vi "String To Variant.vi"(4 "Type Enum [auto]":T1, 5 "Strip Whitespace? [T]":bool=TRUE, 6 "Variant Type\\default":variant, 7 "Name (error)":string, 8 "error in (no error)":errorcluster, 9 "Use LV Default? [F]":bool, 10 "String":string, 11 "Registry Object":refnum<class "Carya Config.lvclass">) -> (0 "error out":errorcluster, 2 "Variant":variant, 3 "Registry Object":refnum<class "Carya Config.lvclass">)   [LabVIEW 2013, in "Carya Config.lvclass"]
doc: "Copyright 2018, Carya Automatisering, Wiebe Walstra."
uses:
  Carya Config.lvclass
  <vilib>/Utility/VariantDataType/Type.ctl
  <vilib>/Utility/error.llb/Error Cluster From Error Code.vi
  <vilib>/ErrorRing/Error Ring.xnode
  <vilib>/Utility/VariantDataType/VariantType.lvlib
  CConfig Variant Accessor/CConfig Variant Accessor.lvclass
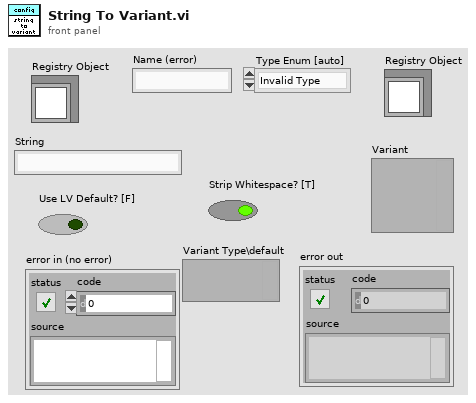
[diagram p1: front panel]
types:
  T1 = typedef "VariantType.lvlib/Type.ctl" = enum8{"Invalid Type", "Void", "I8", "I16", "I32", "I64", "U8", "U16", "U32", "U64", "Single Float", "Double Float", "Extended Float", "Single Complex", "Double Complex", "Extended Complex", "Enum U8", "Enum U16", "Enum U32", "Enum U64", "Single Float With Unit", "Double Float With Unit", "Extended Float With Unit", "Single Complex with Unit", "Double Complex with Unit", "Extended Complex with Unit", "Boolean", "String", "Path", "Picture", "Tag", "Array", "Cluster", "Variant", "LV Variant", "Waveform", "Timestamp", "Digital Waveform", "Digital Data", "ExpressData", "Refnum", "External Data", "VI", "Poly VI", "LabVIEW Class Instance", "Fixed Point"}
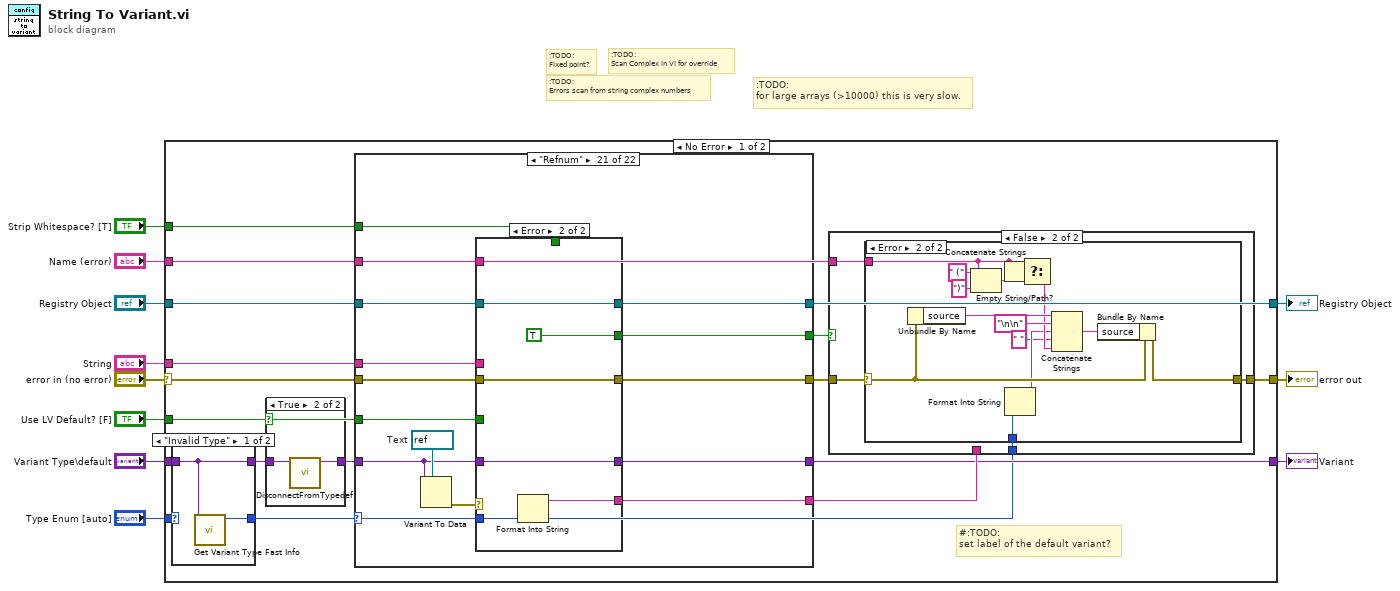
[diagram p0: block diagram]
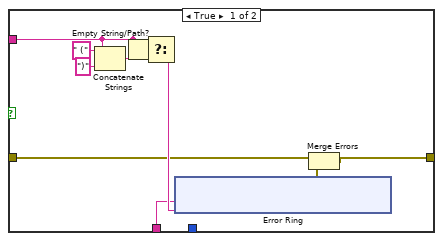
[diagram p2: hidden frame]
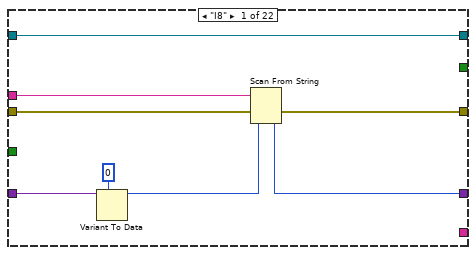
[diagram p6: hidden frame]
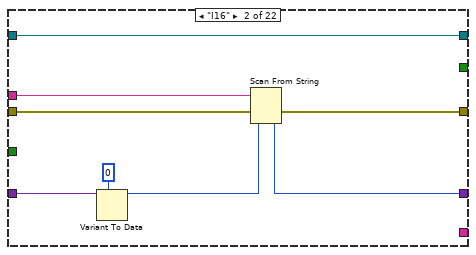
[diagram p7: hidden frame]
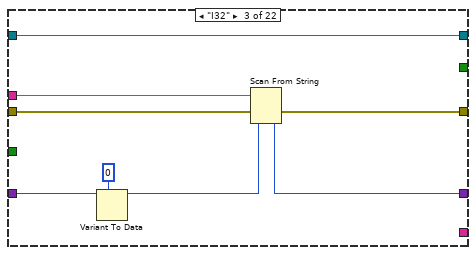
[diagram p8: hidden frame]
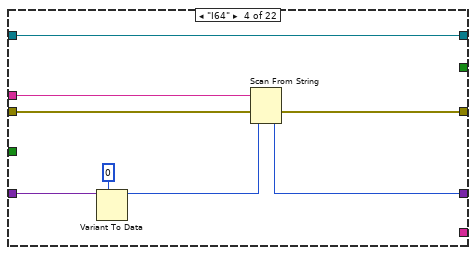
[diagram p9: hidden frame]
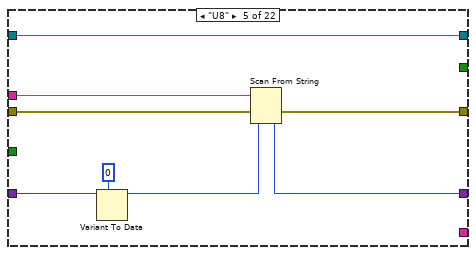
[diagram p10: hidden frame]
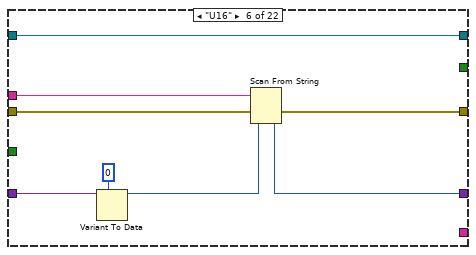
[diagram p11: hidden frame]
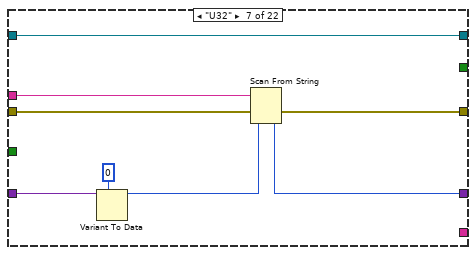
[diagram p12: hidden frame]
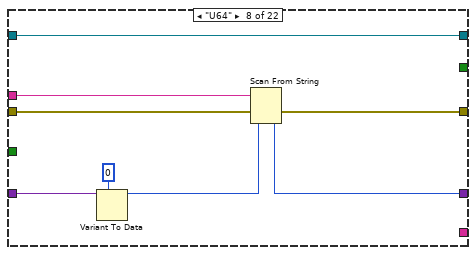
[diagram p13: hidden frame]
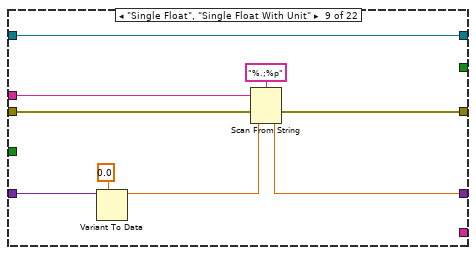
[diagram p14: hidden frame]
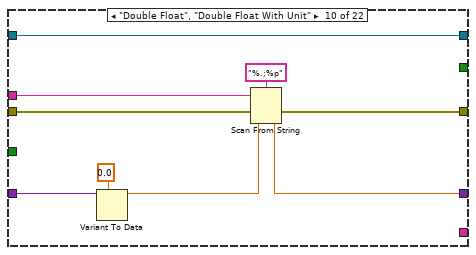
[diagram p15: hidden frame]
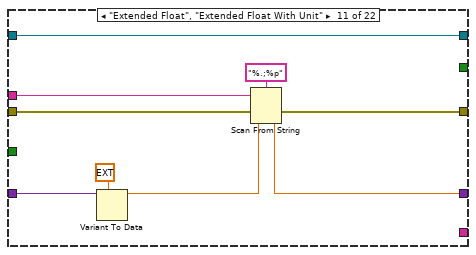
[diagram p16: hidden frame]
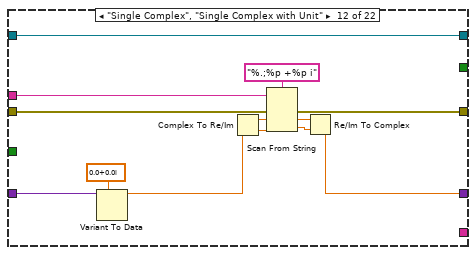
[diagram p17: hidden frame]
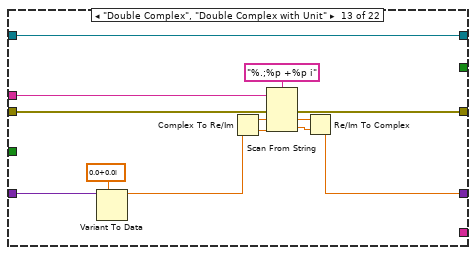
[diagram p18: hidden frame]
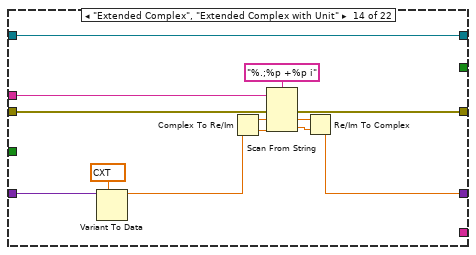
[diagram p19: hidden frame]
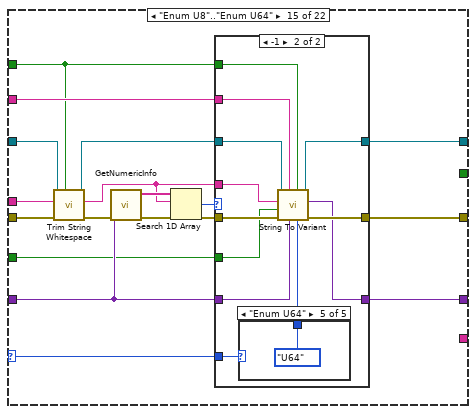
[diagram p20: hidden frame]
diagram:
  # ":TODO:\nfor large arrays (>10000) this is very slow."
  # ":TODO:\nScan Complex in VI for override"
  # ":TODO:\nErrors scan from string complex numbers"
  # ":TODO:\nFixed point?"
  n1 = case shown="No Error" "error in (no error)" {
    selector: "error in (no error)" -> [w15 w648]
    tunnel: "String" -> [w12 _]
    tunnel: "Registry Object" -> [w28 w649]
    tunnel: [w27 w649] -> w9
    tunnel: "Type Enum [auto]" -> [w26 _]
    tunnel: "Strip Whitespace? [T]" -> [w23 _]
    tunnel: "Name (error)" -> [w21 _]
    tunnel: "Use LV Default? [F]" -> [w18 _]
    tunnel: "Variant Type\\default" -> [w17 w647]
    tunnel: [w16 w647] -> w3
    tunnel: [w14 w648] -> w1
    frame No Error {
      # "#:TODO:\nset label of the default variant?"
      n2 = case shown="\"Invalid Type\"" w26 {
        selector: w26 -> [_ w72]
        tunnel: w17 -> [w69 w71]
        tunnel: [w70 w72] -> w13
        tunnel: [w69 w71] -> w24
        frame "Invalid Type" {
          n3 = call "Get Variant Type Fast Info.vi"("Variant"=w69) -> ("Type Enum"=w70:T1)  [unwired: 6 in, 4 out]
        }
        frame Default {
        }
      }
      n4 = case shown="True" w18 {
        tunnel: [w66 w68] -> w25
        tunnel: w24 -> [w66 w67]
        frame False {
        }
        frame True {
          n5 = call <vilib>:"DisconnectFromTypedef.vi"("lvvar in"=w67) -> ("lvvar out"=w68:variant)  [unwired: 4 in, 1 out]
        }
      }
      n6 = case shown="\"Refnum\"" w13 {
        selector: w13 -> [_ _ _ _ _ _ _ _ _ _ _ _ _ _ w210 _ _ _ _ _ w622 w642]
        tunnel: [w78 w86 w94 w102 w109 w117 w125 w133 w143 w151 w160 w173 w186 w199 w216 w257 w285 w293 w307 w605 w617 w645] -> w22
        tunnel: w15 -> [w74 w82 w90 w98 w110 w118 w126 w134 w140 w152 w161 w174 w187 w200 w218 w260 w287 w294 w308 w608 w618 w645]
        tunnel: w25 -> [w80 w88 w96 w104 w112 w120 w128 w136 w145 w154 w163 w176 w189 w202 w213 w263 _ w296 w305 _ w616 w646]
        tunnel: w21 -> [_ _ _ _ _ _ _ _ _ _ _ _ _ _ w215 _ _ _ w306 _ w610 _]
        tunnel: [w76 w84 w92 w100 w107 w115 w123 w131 w141 w149 w158 w172 w177 w190 w212 w259 w275 w288 w303 w607 w615 w646] -> w16
        tunnel: w12 -> [w75 w83 w91 w99 w106 w114 w122 w130 w139 w148 w157 w170 w184 w197 w206 w256 w283 w292 w302 w604 w612 _]
        tunnel: w28 -> [w73 w81 w89 w97 w105 w113 w121 w129 w138 w147 w156 w169 w183 w196 w208 w261 w282 w291 w301 w603 w614 w644]
        tunnel: [w73 w81 w89 w97 w105 w113 w121 w129 w138 w147 w156 w169 w183 w196 w214 w261 w286 w290 w300 w606 w613 w644] -> w27
        tunnel: w23 -> [_ _ _ _ _ _ _ _ _ _ _ _ _ _ w204 _ w276 _ w298 _ w609 _]
        tunnel: [_ _ _ _ _ _ _ _ _ _ _ _ _ _ _ _ _ _ _ _ w623 TRUE] -> w20
        tunnel: [_ _ _ _ _ _ _ _ _ _ _ _ _ _ _ _ _ _ _ _ w621 w641] -> w19
        tunnel: w18 -> [_ _ _ _ _ _ _ _ _ _ _ _ _ _ w203 _ _ _ w297 _ w611 _]
        frame "I8" {
          n7 = Variant To Data(type=i8 0, Variant=w80) -> (data=w77:i8)  [unwired: 1 in, 1 out]
          n8 = Scan From String(input string=w75, error in=w74, default 1=w77) -> (error out=w78:errorcluster, output 1=w76:i8)  [unwired: 2 in, 2 out]
        }
        frame "I16" {
          n9 = Variant To Data(type=i16 0, Variant=w88) -> (data=w85:i16)  [unwired: 1 in, 1 out]
          n10 = Scan From String(input string=w83, error in=w82, default 1=w85) -> (error out=w86:errorcluster, output 1=w84:i16)  [unwired: 2 in, 2 out]
        }
        frame "I32" {
          n11 = Variant To Data(type=0, Variant=w96) -> (data=w93:i32)  [unwired: 1 in, 1 out]
          n12 = Scan From String(input string=w91, error in=w90, default 1=w93) -> (error out=w94:errorcluster, output 1=w92:i32)  [unwired: 2 in, 2 out]
        }
        frame "I64" {
          n13 = Variant To Data(type=i64 0, Variant=w104) -> (data=w101:i64)  [unwired: 1 in, 1 out]
          n14 = Scan From String(input string=w99, error in=w98, default 1=w101) -> (error out=w102:errorcluster, output 1=w100:i64)  [unwired: 2 in, 2 out]
        }
        frame "U8" {
          n15 = Variant To Data(type=u8 0, Variant=w112) -> (data=w108:u8)  [unwired: 1 in, 1 out]
          n16 = Scan From String(input string=w106, error in=w110, default 1=w108) -> (error out=w109:errorcluster, output 1=w107:u8)  [unwired: 2 in, 2 out]
        }
        frame "U16" {
          n17 = Variant To Data(type=u16 0, Variant=w120) -> (data=w116:u16)  [unwired: 1 in, 1 out]
          n18 = Scan From String(input string=w114, error in=w118, default 1=w116) -> (error out=w117:errorcluster, output 1=w115:u16)  [unwired: 2 in, 2 out]
        }
        frame "U32" {
          n19 = Variant To Data(type=u32 0, Variant=w128) -> (data=w124:u32)  [unwired: 1 in, 1 out]
          n20 = Scan From String(input string=w122, error in=w126, default 1=w124) -> (error out=w125:errorcluster, output 1=w123:u32)  [unwired: 2 in, 2 out]
        }
        frame "U64" {
          n21 = Variant To Data(type=u64 0, Variant=w136) -> (data=w132:u64)  [unwired: 1 in, 1 out]
          n22 = Scan From String(input string=w130, error in=w134, default 1=w132) -> (error out=w133:errorcluster, output 1=w131:u64)  [unwired: 2 in, 2 out]
        }
        frame "Single Float", "Single Float With Unit" {
          n23 = Variant To Data(type=sgl 0.0, Variant=w145) -> (data=w142:sgl)  [unwired: 1 in, 1 out]
          n24 = Scan From String(format string="%.;%p", input string=w139, error in=w140, default 1=w142) -> (error out=w143:errorcluster, output 1=w141:sgl)  [unwired: 1 in, 2 out]
        }
        frame "Double Float", "Double Float With Unit" {
          n25 = Variant To Data(type=0.0, Variant=w154) -> (data=w150:dbl)  [unwired: 1 in, 1 out]
          n26 = Scan From String(format string="%.;%p", input string=w148, error in=w152, default 1=w150) -> (error out=w151:errorcluster, output 1=w149:dbl)  [unwired: 1 in, 2 out]
        }
        frame "Extended Float", "Extended Float With Unit" {
          n27 = Variant To Data(type=ext 0.0, Variant=w163) -> (data=w159:ext)  [unwired: 1 in, 1 out]
          n28 = Scan From String(format string="%.;%p", input string=w157, error in=w161, default 1=w159) -> (error out=w160:errorcluster, output 1=w158:ext)  [unwired: 1 in, 2 out]
        }
        frame "Single Complex", "Single Complex with Unit" {
          n29 = Variant To Data(type=csg 0.0+0.0i, Variant=w176) -> (data=w171:csg)  [unwired: 1 in, 1 out]
          n30 = Complex To Re/Im(x + iy=w171) -> (x=w167:sgl, y=w166:sgl)
          n31 = Scan From String(format string="%.;%p +%p i", input string=w170, error in=w174, default 1=w167, default 2=w166) -> (error out=w173:errorcluster, output 1=w165:sgl, output 2=w164:sgl)  [unwired: 1 in, 2 out]
          n32 = Re/Im To Complex(1:w164, 2:w165) -> (0:w172:csg)
        }
        frame "Double Complex", "Double Complex with Unit" {
          n33 = Variant To Data(type=cdb 0.0+0.0i, Variant=w189) -> (data=w185:cdb)  [unwired: 1 in, 1 out]
          n34 = Complex To Re/Im(x + iy=w185) -> (x=w181:dbl, y=w180:dbl)
          n35 = Scan From String(format string="%.;%p +%p i", input string=w184, error in=w187, default 1=w181, default 2=w180) -> (error out=w186:errorcluster, output 1=w179:dbl, output 2=w178:dbl)  [unwired: 1 in, 2 out]
          n36 = Re/Im To Complex(1:w178, 2:w179) -> (0:w177:cdb)
        }
        frame "Extended Complex", "Extended Complex with Unit" {
          n37 = Variant To Data(type=cxt 0.0+0.0i, Variant=w202) -> (data=w198:cxt)  [unwired: 1 in, 1 out]
          n38 = Complex To Re/Im(x + iy=w198) -> (x=w194:ext, y=w193:ext)
          n39 = Scan From String(format string="%.;%p +%p i", input string=w197, error in=w200, default 1=w194, default 2=w193) -> (error out=w199:errorcluster, output 1=w192:ext, output 2=w191:ext)  [unwired: 1 in, 2 out]
          n40 = Re/Im To Complex(1:w191, 2:w192) -> (0:w190:cxt)
        }
        frame "Enum U8".."Enum U64" {
          n41 = call-dynamic "Trim String Whitespace.vi"("Strip Whitespace? [T]"=w204, "error in (no error)"=w218, "String"=w206, "Registry Object"=w208) -> ("error out"=w209:errorcluster, "Trimmed string"=w205:string, "Registry Object"=w207:refnum<class "Carya Config.lvclass">)  [unwired: 5 in]
          n42 = call <vilib>:"GetNumericInfo.vi"("error in (no error)"=w209, "Variant"=w213) -> ("error out"=w217:errorcluster, "EnumNames"=w219:string[])  [unwired: 6 in, 2 out]
          n43 = Search 1D Array(1D array=w219, element=w205) -> (index of element=w211:i32)  [unwired: 1 in]
          n44 = case shown="-1" w211 {
            selector: w211 -> [w222 _]
            tunnel: w217 -> [w223 w249]
            tunnel: [w223 w248] -> w216
            tunnel: w215 -> [_ w247]
            tunnel: w207 -> [w224 w246]
            tunnel: [w224 w245] -> w214
            tunnel: w213 -> [_ w244]
            tunnel: [w221 w243] -> w212
            tunnel: w205 -> [_ w242]
            tunnel: w210 -> [w220 w241]
            tunnel: w204 -> [_ w239]
            tunnel: w203 -> [_ w238]
            frame Default {
              n45 = case shown="\"Enum U8\"" w220 {
                tunnel: w222 -> [_ w228 w231 w234 w237]
                tunnel: [variant ("lvvar out") w227 w230 w233 w236] -> w221
                frame Default {
                }
                frame "Enum U8" {
                  n46 = Variant To Data(type=u8 0, Variant=w228) -> (data=w227:u8)  [unwired: 1 in, 1 out]
                }
                frame "Enum U16" {
                  n47 = Variant To Data(type=u16 0, Variant=w231) -> (data=w230:u16)  [unwired: 1 in, 1 out]
                }
                frame "Enum U32" {
                  n48 = Variant To Data(type=u32 0, Variant=w234) -> (data=w233:u32)  [unwired: 1 in, 1 out]
                }
                frame "Enum U64" {
                  n49 = Variant To Data(type=u64 0, Variant=w237) -> (data=w236:u64)  [unwired: 1 in, 1 out]
                }
              }
            }
            frame -1 {
              n50 = case shown="\"Enum U64\"" w241 {
                tunnel: [_ Type."U8" ("Type Enum [auto]") Type."U16" ("Type Enum [auto]") Type."U32" ("Type Enum [auto]") Type."U64" ("Type Enum [auto]")] -> w240
                frame Default {
                }
                frame "Enum U8" {
                }
                frame "Enum U16" {
                }
                frame "Enum U32" {
                }
                frame "Enum U64" {
                }
              }
              n51 = call-dynamic "String To Variant.vi"("Type Enum [auto]"=w240, "Strip Whitespace? [T]"=w239, "Variant Type\\default"=w244, "Name (error)"=w247, "error in (no error)"=w249, "Use LV Default? [F]"=w238, "String"=w242, "Registry Object"=w246) -> ("error out"=w248:errorcluster, "Variant"=w243:variant, "Registry Object"=w245:refnum<class "Carya Config.lvclass">)  [unwired: 1 in]
            }
          }
        }
        frame "Boolean" {
          # "false, true\nF, T\nFALSE, TRUE\n0, 1\nY, N\nYes, No\nYES, NO"
          n52 = Variant To Data(type=TRUE, Variant=w263) -> (data=w258:bool)  [unwired: 1 in, 1 out]
          n53 = Decimal String To Number(string=w256, default (0L)=0 ("default (0 I32)")) -> (offset past number=w254:i32)  [unwired: 1 in, 1 out]
          n54 = case shown="1.." w254 {
            tunnel: w260 -> [w269 w274]
            tunnel: [w268 w273] -> w259
            tunnel: w258 -> [w267 w272]
            tunnel: [w266 w271] -> w257
            tunnel: w256 -> [w265 w270]
            frame 1.. {
              n55 = Scan From String(format string="%d", input string=w265, error in=w269, default 1=w267) -> (error out=w266:errorcluster, output 1=w268:bool)  [unwired: 1 in, 2 out]
            }
            frame Default {
              n56 = Scan From String(input string=w270, error in=w274, default 1=w272) -> (error out=w271:errorcluster, output 1=w273:bool)  [unwired: 2 in, 2 out]
            }
          }
        }
        frame "String" {
          n57 = call-dynamic "String (RAW) To String.vi"("error in (no error)"=w287, "String (RAW)"=w283, "Registry Object"=w282) -> ("error out"=w284:errorcluster, "String"=w278:string, "Registry Object"=w280:refnum<class "Carya Config.lvclass">)  [unwired: 6 in]
          n58 = call-dynamic "Trim String Whitespace.vi"("Strip Whitespace? [T]"=w276, "error in (no error)"=w284, "String"=w278, "Registry Object"=w280) -> ("error out"=w281:errorcluster, "Trimmed string"=w277:string, "Registry Object"=w279:refnum<class "Carya Config.lvclass">)  [unwired: 5 in]
          n59 = call-dynamic "Unescape String.vi"("error in (no error)"=w281, "String"=w277, "Registry Object"=w279) -> ("error out"=w285:errorcluster, "Unescaped string"=w275:string, "Registry Object"=w286:refnum<class "Carya Config.lvclass">)  [unwired: 6 in]
        }
        frame "Path" {
          n60 = Variant To Data(type=path "", Variant=w296) -> (data=w289:path)  [unwired: 1 in, 1 out]
          n61 = call-dynamic "String To Path.vi"("Default"=w289, "error in (no error)"=w294, "String"=w292, "Registry Object"=w291) -> ("error out"=w293:errorcluster, "Path"=w288:path, "Registry Object"=w290:refnum<class "Carya Config.lvclass">)  [unwired: 5 in]
        }
        frame "Array" {
          n62 = call <vilib>:"GetArrayInfo.vi"("Variant"=w305) -> ("ArrayElement"=w299:variant, "NDims"=w304:i32)  [unwired: 7 in, 2 out]
          n63 = case shown="1" w304 {
            selector: w304 -> [w314 _]
            tunnel: w308 -> [w315 w332]
            tunnel: [w312 w335] -> w307
            tunnel: w306 -> [w313 w329]
            tunnel: w305 -> [w309 w327]
            tunnel: [w309 w334] -> w303
            tunnel: w302 -> [_ w333]
            tunnel: w301 -> [w310 w331]
            tunnel: [w310 w330] -> w300
            tunnel: w299 -> [_ w326]
            tunnel: w298 -> [_ w325]
            tunnel: w297 -> [_ w324]
            frame Default {
              n64 = xnode "Error Ring"("parameter 0"=w314, "parameter 1"=w313) -> ("error out"=w311:errorcluster)
              n65 = Merge Errors(w315, w311) -> (w312:errorcluster)
            }
            frame 1 {
              n66 = call "Get Variant Type Fast Info.vi"("Variant"=w326) -> ("Type Enum"=w328:T1)  [unwired: 6 in, 4 out]
              n67 = case shown="Default" w328 {
                selector: w328 -> [_ _ _ _ _ _ _ _ _ _ _ _ _ w586]
                tunnel: [w336 w355 w374 w393 w412 w431 w450 w469 w494 w500 w519 w538 w558 w583] -> w335
                tunnel: [w346 w365 w384 w403 w422 w441 w460 w479 w497 w510 w529 w548 w557 w581] -> w334
                tunnel: w333 -> [w344 w363 w382 w401 w420 w439 w458 w477 w488 w508 w527 w546 w561 w576]
                tunnel: w332 -> [w337 w356 w375 w394 w413 w432 w451 w470 w495 w501 w520 w539 w560 w589]
                tunnel: w331 -> [w345 w364 w383 w402 w421 w440 w459 w478 w493 w509 w528 w547 w562 w574]
                tunnel: [w345 w364 w383 w402 w421 w440 w459 w478 w492 w509 w528 w547 w562 w570] -> w330
                tunnel: w329 -> [_ _ _ _ _ _ _ _ _ _ _ _ _ w588]
                tunnel: w326 -> [_ _ _ _ _ _ _ _ _ _ _ _ _ w587]
                tunnel: w327 -> [w347 w366 w385 w404 w423 w442 w461 w480 w498 w511 w530 w549 w557 w584]
                tunnel: w325 -> [_ _ _ _ _ _ _ _ w491 _ _ _ _ w573]
                tunnel: w324 -> [_ _ _ _ _ _ _ _ _ _ _ _ _ w572]
                frame "I8" {
                  # "we can't use spr. str to array directly to get the type...\nwe'll not notice any errors..."
                  n68 = Spreadsheet String To Array(delimiter (Tab)=",", format string="", spreadsheet string=w344, array type (2D Dbl)=string[] []) -> (array=w340:string[])
                  n69 = for {
                    tunnel: w340 -> [w354] mode=indexing
                    tunnel: [w351] -> w339 mode=indexing
                    shift-right: [w349] -> w336
                    shift-left: w337 -> [w350]
                    n70 = Scan From String(format string="%d", input string=w354, error in=w350, default 1=i8 0 ("default value 1")) -> (error out=w349:errorcluster, output 1=w351:i8)  [unwired: 1 in, 2 out]
                  }
                  n71 = Variant To Flattened String(Variant=w347) -> (1:w348:i16[])  [unwired: 1 out]
                  n72 = Flatten To String(anything=w339) -> (data string=w338:string)  [unwired: 3 in, 2 out]
                  n73 = Flattened String To Variant(6:w338, 7:w348) -> (3:w346:variant)  [unwired: 1 in, 1 out]
                }
                frame "I16" {
                  # "we can't use spr. str to array directly to get the type...\nwe'll not notice any errors..."
                  n74 = Spreadsheet String To Array(delimiter (Tab)=",", format string="", spreadsheet string=w363, array type (2D Dbl)=string[] []) -> (array=w359:string[])
                  n75 = for {
                    tunnel: w359 -> [w373] mode=indexing
                    tunnel: [w370] -> w358 mode=indexing
                    shift-right: [w368] -> w355
                    shift-left: w356 -> [w369]
                    n76 = Scan From String(format string="%d", input string=w373, error in=w369, default 1=i16 0 ("default value 1")) -> (error out=w368:errorcluster, output 1=w370:i16)  [unwired: 1 in, 2 out]
                  }
                  n77 = Variant To Flattened String(Variant=w366) -> (1:w367:i16[])  [unwired: 1 out]
                  n78 = Flatten To String(anything=w358) -> (data string=w357:string)  [unwired: 3 in, 2 out]
                  n79 = Flattened String To Variant(6:w357, 7:w367) -> (3:w365:variant)  [unwired: 1 in, 1 out]
                }
                frame "I32" {
                  # "we can't use spr. str to array directly to get the type...\nwe'll not notice any errors..."
                  n80 = Spreadsheet String To Array(delimiter (Tab)=",", format string="", spreadsheet string=w382, array type (2D Dbl)=string[] []) -> (array=w378:string[])
                  n81 = for {
                    tunnel: w378 -> [w392] mode=indexing
                    tunnel: [w389] -> w377 mode=indexing
                    shift-right: [w387] -> w374
                    shift-left: w375 -> [w388]
                    n82 = Scan From String(format string="%d", input string=w392, error in=w388, default 1=0 ("default value 1")) -> (error out=w387:errorcluster, output 1=w389:i32)  [unwired: 1 in, 2 out]
                  }
                  n83 = Variant To Flattened String(Variant=w385) -> (1:w386:i16[])  [unwired: 1 out]
                  n84 = Flatten To String(anything=w377) -> (data string=w376:string)  [unwired: 3 in, 2 out]
                  n85 = Flattened String To Variant(6:w376, 7:w386) -> (3:w384:variant)  [unwired: 1 in, 1 out]
                }
                frame "I64" {
                  # "we can't use spr. str to array directly to get the type...\nwe'll not notice any errors..."
                  n86 = Spreadsheet String To Array(delimiter (Tab)=",", format string="", spreadsheet string=w401, array type (2D Dbl)=string[] []) -> (array=w397:string[])
                  n87 = for {
                    tunnel: w397 -> [w411] mode=indexing
                    tunnel: [w408] -> w396 mode=indexing
                    shift-right: [w406] -> w393
                    shift-left: w394 -> [w407]
                    n88 = Scan From String(format string="%d", input string=w411, error in=w407, default 1=i64 0 ("default value 1")) -> (error out=w406:errorcluster, output 1=w408:i64)  [unwired: 1 in, 2 out]
                  }
                  n89 = Variant To Flattened String(Variant=w404) -> (1:w405:i16[])  [unwired: 1 out]
                  n90 = Flatten To String(anything=w396) -> (data string=w395:string)  [unwired: 3 in, 2 out]
                  n91 = Flattened String To Variant(6:w395, 7:w405) -> (3:w403:variant)  [unwired: 1 in, 1 out]
                }
                frame "U8" {
                  # "we can't use spr. str to array directly to get the type...\nwe'll not notice any errors..."
                  n92 = Spreadsheet String To Array(delimiter (Tab)=",", format string="", spreadsheet string=w420, array type (2D Dbl)=string[] []) -> (array=w416:string[])
                  n93 = for {
                    tunnel: w416 -> [w430] mode=indexing
                    tunnel: [w427] -> w415 mode=indexing
                    shift-right: [w425] -> w412
                    shift-left: w413 -> [w426]
                    n94 = Scan From String(format string="%d", input string=w430, error in=w426, default 1=u8 0 ("default value 1")) -> (error out=w425:errorcluster, output 1=w427:u8)  [unwired: 1 in, 2 out]
                  }
                  n95 = Variant To Flattened String(Variant=w423) -> (1:w424:i16[])  [unwired: 1 out]
                  n96 = Flatten To String(anything=w415) -> (data string=w414:string)  [unwired: 3 in, 2 out]
                  n97 = Flattened String To Variant(6:w414, 7:w424) -> (3:w422:variant)  [unwired: 1 in, 1 out]
                }
                frame "U16" {
                  # "we can't use spr. str to array directly to get the type...\nwe'll not notice any errors..."
                  n98 = Spreadsheet String To Array(delimiter (Tab)=",", format string="", spreadsheet string=w439, array type (2D Dbl)=string[] []) -> (array=w435:string[])
                  n99 = for {
                    tunnel: w435 -> [w449] mode=indexing
                    tunnel: [w446] -> w434 mode=indexing
                    shift-right: [w444] -> w431
                    shift-left: w432 -> [w445]
                    n100 = Scan From String(format string="%d", input string=w449, error in=w445, default 1=u16 0 ("default value 1")) -> (error out=w444:errorcluster, output 1=w446:u16)  [unwired: 1 in, 2 out]
                  }
                  n101 = Variant To Flattened String(Variant=w442) -> (1:w443:i16[])  [unwired: 1 out]
                  n102 = Flatten To String(anything=w434) -> (data string=w433:string)  [unwired: 3 in, 2 out]
                  n103 = Flattened String To Variant(6:w433, 7:w443) -> (3:w441:variant)  [unwired: 1 in, 1 out]
                }
                frame "U32" {
                  # "we can't use spr. str to array directly to get the type...\nwe'll not notice any errors..."
                  n104 = Spreadsheet String To Array(delimiter (Tab)=",", format string="", spreadsheet string=w458, array type (2D Dbl)=string[] []) -> (array=w454:string[])
                  n105 = for {
                    tunnel: w454 -> [w468] mode=indexing
                    tunnel: [w465] -> w453 mode=indexing
                    shift-right: [w463] -> w450
                    shift-left: w451 -> [w464]
                    n106 = Scan From String(format string="%d", input string=w468, error in=w464, default 1=u32 0 ("default value 1")) -> (error out=w463:errorcluster, output 1=w465:u32)  [unwired: 1 in, 2 out]
                  }
                  n107 = Variant To Flattened String(Variant=w461) -> (1:w462:i16[])  [unwired: 1 out]
                  n108 = Flatten To String(anything=w453) -> (data string=w452:string)  [unwired: 3 in, 2 out]
                  n109 = Flattened String To Variant(6:w452, 7:w462) -> (3:w460:variant)  [unwired: 1 in, 1 out]
                }
                frame "U64" {
                  # "we can't use spr. str to array directly to get the type...\nwe'll not notice any errors..."
                  n110 = Spreadsheet String To Array(delimiter (Tab)=",", format string="", spreadsheet string=w477, array type (2D Dbl)=string[] []) -> (array=w473:string[])
                  n111 = for {
                    tunnel: w473 -> [w487] mode=indexing
                    tunnel: [w484] -> w472 mode=indexing
                    shift-right: [w482] -> w469
                    shift-left: w470 -> [w483]
                    n112 = Scan From String(format string="%d", input string=w487, error in=w483, default 1=u64 0 ("default value 1")) -> (error out=w482:errorcluster, output 1=w484:u64)  [unwired: 1 in, 2 out]
                  }
                  n113 = Variant To Flattened String(Variant=w480) -> (1:w481:i16[])  [unwired: 1 out]
                  n114 = Flatten To String(anything=w472) -> (data string=w471:string)  [unwired: 3 in, 2 out]
                  n115 = Flattened String To Variant(6:w471, 7:w481) -> (3:w479:variant)  [unwired: 1 in, 1 out]
                }
                frame "String" {
                  # "we can't use spr. str to array directly to get the type...\nwe'll not notice any errors..."
                  n116 = call-dynamic "String To Array.vi"("Unescape? [F]"=TRUE, "Strip Whitespace? [T]"=w491, "error in (no error)"=w495, "resulting string"=w488, "Registry Object"=w493) -> ("error out"=w494:errorcluster, "Array"=w489:string[], "Registry Object"=w492:refnum<class "Carya Config.lvclass">)  [unwired: 4 in]
                  n117 = Variant To Flattened String(Variant=w498) -> (1:w499:i16[])  [unwired: 1 out]
                  n118 = Flatten To String(anything=w489) -> (data string=w496:string)  [unwired: 3 in, 2 out]
                  n119 = Flattened String To Variant(6:w496, 7:w499) -> (3:w497:variant)  [unwired: 1 in, 1 out]
                }
                frame "Single Float", "Single Float With Unit" {
                  # "we can't use spr. str to array directly to get the type...\nwe'll not notice any errors..."
                  n120 = Spreadsheet String To Array(delimiter (Tab)=",", format string="", spreadsheet string=w508, array type (2D Dbl)=string[] []) -> (array=w504:string[])
                  n121 = for {
                    tunnel: w504 -> [w518] mode=indexing
                    tunnel: [w515] -> w503 mode=indexing
                    shift-right: [w513] -> w500
                    shift-left: w501 -> [w514]
                    n122 = Scan From String(format string="%.;%p", input string=w518, error in=w514, default 1=sgl 0.0 ("default value 1")) -> (error out=w513:errorcluster, output 1=w515:sgl)  [unwired: 1 in, 2 out]
                  }
                  n123 = Variant To Flattened String(Variant=w511) -> (1:w512:i16[])  [unwired: 1 out]
                  n124 = Flatten To String(anything=w503) -> (data string=w502:string)  [unwired: 3 in, 2 out]
                  n125 = Flattened String To Variant(6:w502, 7:w512) -> (3:w510:variant)  [unwired: 1 in, 1 out]
                }
                frame "Double Float", "Double Float With Unit" {
                  # "we can't use spr. str to array directly to get the type...\nwe'll not notice any errors..."
                  n126 = Spreadsheet String To Array(delimiter (Tab)=",", format string="", spreadsheet string=w527, array type (2D Dbl)=string[] []) -> (array=w523:string[])
                  n127 = for {
                    tunnel: w523 -> [w537] mode=indexing
                    tunnel: [w534] -> w522 mode=indexing
                    shift-right: [w532] -> w519
                    shift-left: w520 -> [w533]
                    n128 = Scan From String(format string="%.;%p", input string=w537, error in=w533, default 1=0.0 ("default value 1")) -> (error out=w532:errorcluster, output 1=w534:dbl)  [unwired: 1 in, 2 out]
                  }
                  n129 = Variant To Flattened String(Variant=w530) -> (1:w531:i16[])  [unwired: 1 out]
                  n130 = Flatten To String(anything=w522) -> (data string=w521:string)  [unwired: 3 in, 2 out]
                  n131 = Flattened String To Variant(6:w521, 7:w531) -> (3:w529:variant)  [unwired: 1 in, 1 out]
                }
                frame "Extended Float", "Extended Float With Unit" {
                  # "we can't use spr. str to array directly to get the type...\nwe'll not notice any errors..."
                  n132 = Spreadsheet String To Array(delimiter (Tab)=",", format string="", spreadsheet string=w546, array type (2D Dbl)=string[] []) -> (array=w542:string[])
                  n133 = for {
                    tunnel: w542 -> [w556] mode=indexing
                    tunnel: [w553] -> w541 mode=indexing
                    shift-right: [w551] -> w538
                    shift-left: w539 -> [w552]
                    n134 = Scan From String(format string="%.;%p", input string=w556, error in=w552, default 1=0.0 ("default value 1")) -> (error out=w551:errorcluster, output 1=w553:dbl)  [unwired: 1 in, 2 out]
                  }
                  n135 = Variant To Flattened String(Variant=w549) -> (1:w550:i16[])  [unwired: 1 out]
                  n136 = Flatten To String(anything=w541) -> (data string=w540:string)  [unwired: 3 in, 2 out]
                  n137 = Flattened String To Variant(6:w540, 7:w550) -> (3:w548:variant)  [unwired: 1 in, 1 out]
                }
                frame "Cluster" {
                  n138 = xnode "Error Ring"("parameter 0"=w561) -> ("error out"=w559:errorcluster)
                  n139 = Merge Errors(w560, w559) -> (w558:errorcluster)
                }
                frame Default {
                  # "for large arrays (>10000) this is very slow."
                  n140 = call-dynamic "String To Array.vi"("error in (no error)"=w589, "resulting string"=w576, "Registry Object"=w574) -> ("error out"=w577:errorcluster, "Array"=w575:string[], "Registry Object"=w571:refnum<class "Carya Config.lvclass">)  [unwired: 6 in]
                  n141 = for {
                    tunnel: w587 -> [w599]
                    tunnel: w575 -> [w596] mode=indexing
                    tunnel: [w594] -> w580 mode=indexing if=w602
                    shift-right: [w600] -> w583
                    shift-left: w577 -> [w601]
                    tunnel: w588 -> [w598]
                    tunnel: w586 -> [w597]
                    tunnel: w573 -> [w590]
                    tunnel: w572 -> [w593]
                    shift-right: [w591] -> w570
                    shift-left: w571 -> [w592]
                    stop <- w600 stop-if-true
                    n142 = call-dynamic "String To Variant.vi"("Type Enum [auto]"=w597, "Strip Whitespace? [T]"=w590, "Variant Type\\default"=w599, "Name (error)"=w598, "error in (no error)"=w601, "Use LV Default? [F]"=w593, "String"=w596, "Registry Object"=w592) -> ("error out"=w600:errorcluster, "Variant"=w595:variant, "Registry Object"=w591:refnum<class "Carya Config.lvclass">)  [unwired: 1 in]
                    n143 = Variant To Flattened String(Variant=w595) -> (data string=w594:string)  [unwired: 1 out]
                    n144 = Not(x=w600) -> (.not. x?=w602:bool)
                  }
                  n145 = Variant To Flattened String(Variant=w584) -> (1:w585:i16[])  [unwired: 1 out]
                  n146 = Array Size(array=w580) -> (size(s)=w579:i32)
                  n147 = Flatten To String(anything=w579) -> (data string=w578:string)  [unwired: 3 in, 2 out]
                  n148 = Concatenate Strings(w578, w580) -> (w582:string)
                  n149 = Flattened String To Variant(6:w582, 7:w585) -> (3:w581:variant)  [unwired: 1 in, 1 out]
                }
              }
            }
          }
        }
        frame "Timestamp" {
          n150 = call-dynamic "String To Timestamp.vi"("error in (no error)"=w608, "String"=w604, "Registry Object"=w603) -> ("error out"=w605:errorcluster, "Unescaped string"=w607:timestamp, "Registry Object"=w606:refnum<class "Carya Config.lvclass">)  [unwired: 6 in]
        }
        frame "Refnum" {
          w620 = refnum<vi> refnum  # Text
          n151 = Variant To Data(type=w620, Variant=w616) -> (error out=w619:errorcluster)  [unwired: 1 in, 1 out]
          n152 = case shown="Error" w619 {
            tunnel: [_ TRUE] -> w623
            tunnel: w622 -> [_ w639]
            tunnel: [_ w638] -> w621
            tunnel: w618 -> [w634 w635]
            tunnel: [w633 w635] -> w617
            tunnel: w616 -> [w632 w637]
            tunnel: [w631 w637] -> w615
            tunnel: w614 -> [w630 w636]
            tunnel: [w629 w636] -> w613
            tunnel: w612 -> [w628 _]
            tunnel: w611 -> [w627 _]
            tunnel: w610 -> [w625 _]
            tunnel: w609 -> [w624 _]
            frame No Error {
              n153 = call-dynamic "String To Variant.vi"("Type Enum [auto]"=Type."String", "Strip Whitespace? [T]"=w624, "Variant Type\\default"=w632, "Name (error)"=w625, "error in (no error)"=w634, "Use LV Default? [F]"=w627, "String"=w628, "Registry Object"=w630) -> ("error out"=w633:errorcluster, "Variant"=w631:variant, "Registry Object"=w629:refnum<class "Carya Config.lvclass">)  [unwired: 1 in]
            }
            frame Error {
              n154 = Format Into String(w639) -> (resulting string=w638:string)  [unwired: 3 in, 1 out]
            }
          }
        }
        frame Default {
          n155 = Format Into String(w642) -> (resulting string=w641:string)  [unwired: 3 in, 1 out]
        }
      }
      n156 = case shown="False" w20 {
        tunnel: w22 -> [w32 w48]
        tunnel: [w31 w50] -> w14
        tunnel: w21 -> [w30 w49]
        tunnel: w19 -> [w29 _]
        tunnel: w13 -> [_ w47]
        frame True {
          n157 = Concatenate Strings(" (" ("string"), w30, ")" ("string")) -> (w37:string)
          n158 = Empty String/Path?(string/path=w30) -> (empty?=w34:bool)
          n159 = Select(t=w30, s=w34, f=w37) -> (s? t:f=w38:string)
          n160 = xnode "Error Ring"("parameter 0"=w29, "parameter 1"=w38) -> ("error out"=w33:errorcluster)
          n161 = Merge Errors(w32, w33) -> (w31:errorcluster)
        }
        frame False {
          n162 = case shown="Error" w48 {
            selector: w48 -> [w51 w60]
            tunnel: [w51 w59] -> w50
            tunnel: w49 -> [_ w61]
            tunnel: w47 -> [_ w54]
            frame No Error {
            }
            frame Error {
              n163 = Unbundle By Name(w60) -> ("source"=w58:string)
              n164 = Concatenate Strings(" (" ("string"), w61, ")" ("string")) -> (w65:string)
              n165 = Empty String/Path?(string/path=w61) -> (empty?=w62:bool)
              n166 = Format Into String(w54) -> (resulting string=w53:string)  [unwired: 3 in, 1 out]
              n167 = Select(t=w61, s=w62, f=w65) -> (s? t:f=w55:string)
              n168 = Concatenate Strings(w58, "\n\n" ("string"), w53, " " ("string"), w55) -> (w57:string)
              n169 = Bundle By Name(cluster=w60, "source"=w57) -> (w59:errorcluster)
            }
          }
        }
      }
    }
    frame Error {
    }
  }
  "Registry Object" <- w9
  "error out" <- w1
  "Variant" <- w3
